vi "Cal BC (VIRef).vi"(8 "error in (no error)":errorcluster, 10 "BC in":variant, 11 "Domain_Steady_2D_Polygon in":refnum<class "NI_Domain_Steady_2D_Polygon.lvclass">) -> (0 "error out":errorcluster, 2 "BC out":variant, 3 "Domain_Steady_2D_Polygon out":refnum<class "NI_Domain_Steady_2D_Polygon.lvclass">)   [LabVIEW 2017, in "NI_PDE.lvlib" / "NI_Domain_Steady_2D_Polygon.lvclass"]
uses:
  <vilib>/gmath/pde.llb/DomainClass/Domain_Steady_2D_Polygon/NI_Domain_Steady_2D_Polygon.lvclass
  <vilib>/gmath/pde.llb/BCClass/BC_Steady_2D_VIRef/BC Data.ctl
  <vilib>/gmath/pde.llb/Common/PDE_BC Type.ctl
  <vilib>/gmath/pde.llb/Common/PDE_BC Position 2D.ctl
  <vilib>/gmath/pde.llb/BCClass/BC_Steady_2D_Numeric/BC Data.ctl
  <vilib>/gmath/pde.llb/DomainClass/Domain_Steady_2D_Polygon/NI_Domain_Steady_2D_Polygon.lvclass/NI_Domain_Steady_2D_Polygon.ctl
  <vilib>/gmath/NI_PDE.lvlib
  <vilib>/gmath/pde.llb/BCClass/BC_Steady_2D_VIRef/NI_BC_Steady_2D_VIRef.lvclass
  <vilib>/gmath/pde.llb/BCClass/BC_Steady_2D_Numeric/NI_BC_Steady_2D_Numeric.lvclass
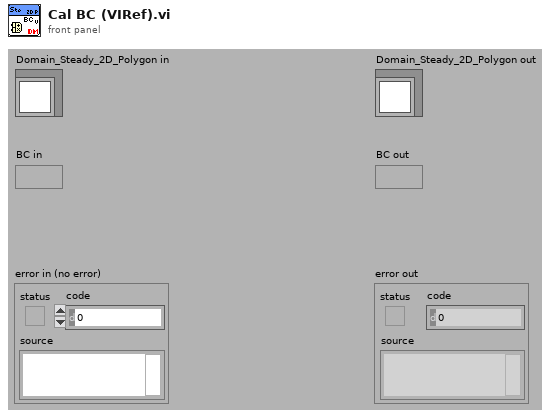
[diagram p1: front panel]
types:
  T1 = typedef "NI_PDE.lvlib/NI_BC_Steady_2D_Numeric.lvclass/BC Data.ctl" = cluster{"type":T2, "position":T3, "G":dbl[]}
  T2 = typedef "NI_PDE.lvlib/PDE_BC Type.ctl" = i32
  T3 = typedef "NI_PDE.lvlib/PDE_BC Position 2D.ctl" = i32
  T4 = typedef "NI_PDE.lvlib/NI_BC_Steady_2D_VIRef.lvclass/BC Data.ctl" = cluster{"type":T2, "position":T3, "G":refnum<vi>, "data":variant}
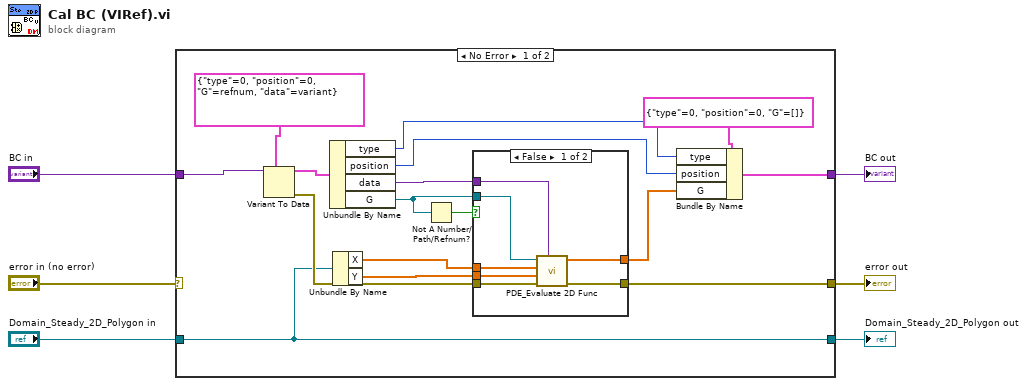
[diagram p0: block diagram]
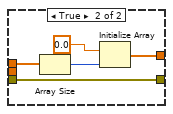
[diagram p2: hidden frame]
diagram:
  n1 = case shown="No Error" "error in (no error)" {
    selector: "error in (no error)" -> [_ w37]
    tunnel: "Domain_Steady_2D_Polygon in" -> [w7 w36]
    tunnel: [w7 w36] -> w6
    tunnel: [w11 w37] -> w5
    tunnel: [w18 w35] -> w2
    tunnel: "BC in" -> [w22 w35]
    frame No Error {
      n2 = Variant To Data(type=T4 {"type"=0, "position"=0, "G"=refnum, "data"=variant} ("BC data"), Variant=w22) -> (data=w20:T4, error out=w8:errorcluster)  [unwired: 1 in]
      n3 = Unbundle By Name(w20) -> ("type"=w17:T2, "position"=w16:T3, "data"=w14:variant, "G"=w13:refnum<vi>)
      n4 = Unbundle By Name(w7) -> ("X"=w10:dbl[], "Y"=w9:dbl[])
      n5 = Not A Number/Path/Refnum?(number/path/refnum=w13) -> (NaN/Path/Refnum?=w15:bool)
      n6 = case shown="False" w15 {
        tunnel: [w25 w34] -> w12
        tunnel: w8 -> [w29 w32]
        tunnel: [w28 w32] -> w11
        tunnel: w13 -> [w27 _]
        tunnel: w14 -> [w26 _]
        tunnel: w10 -> [w24 w30]
        tunnel: w9 -> [w23 _]
        frame False {
          n7 = call <vilib>:"PDE_Evaluate 2D Func.vi"("data"=w26, "error in (no error)"=w29, "Y"=w23, "X"=w24, "VIRef"=w27) -> ("error out"=w28:errorcluster, "F(x, y)"=w25:dbl[])  [unwired: 5 out]
        }
        frame True {
          n8 = Array Size(array=w30) -> (size(s)=w31:i32)
          n9 = Initialize Array(0.0 ("element"), w31) -> (w34:dbl[])
        }
      }
      n10 = Bundle By Name(cluster=T1 {"type"=0, "position"=0, "G"=[]} ("BC data"), "type"=w17, "position"=w16, "G"=w12) -> (w18:T1)
    }
    frame Error {
    }
  }
  "Domain_Steady_2D_Polygon out" <- w6
  "error out" <- w5
  "BC out" <- w2
